vi "Wrap Data for UI Update.vi"(1 "References":T3, 2 "fpga inteface in":refnum<k20>, 3 "image metadata":T2={"serial channel"=0.0, "frame number"=0, "data type"=enum."Frame Start", "width"=0, "height"=0, "image bytes"=0, "total bytes"=0, "little endian"=FALSE, "Status"="Ready for Acquisition"}, 4 "Active Channel":string, 5 "error in":errorcluster) -> (7 "State message":string, 10 "Acqusition In Progress":bool, 11 "status":bool, 12 "Acquisition Duration":dbl, 14 "Image Data":string, 15 "Bytes Acquired":u64, 16 "PowerOverCoaxCurrent":dbl, 17 "PowerOverCoaxVoltage":dbl, 18 "width":u64, 19 "height":u64)   [LabVIEW 2025, in "Automotive Vision.lvclass"]
doc: "Wrap data for the measurement results cluster."
uses:
  Automotive Vision.lvclass
  Automotive Vision.lvclass/Automotive Vision.ctl
  <instrlib>/FlexRIO/CSI-2/v2/Common/Types/LLP Data Type.ctl
  <instrlib>/FlexRIO/CSI-2/v2/Common/NI CSI-2 API Common v2.lvlib
  <resource>/objmgr/niflexrioapiChannel.rc
  <instrlib>/FlexRIO/API/Host/v1/NI FlexRIO API v1.lvlib
  <instrlib>/FlexRIO/API/Host/v1/NI FlexRIO/API/Get Property Reference - Fpga Small.vi
panel:
  out "error out":errorcluster
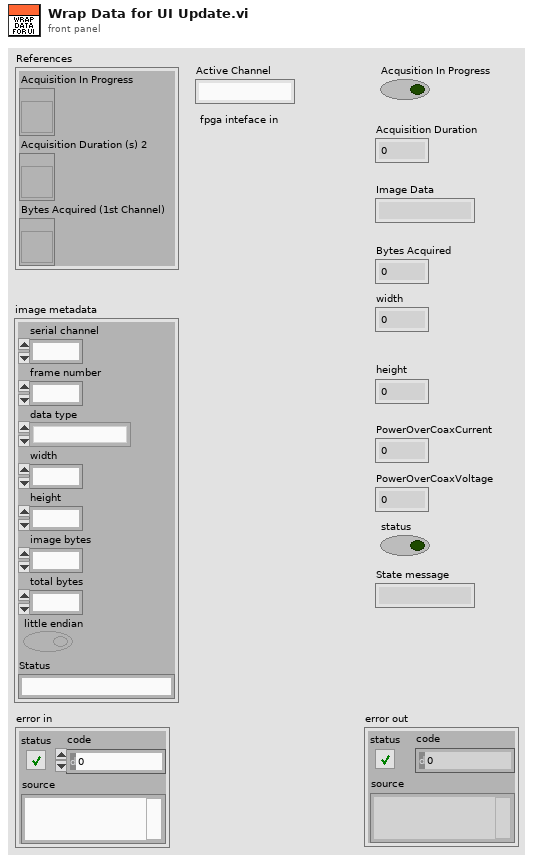
[diagram p1: front panel]
types:
  T1 = typedef "NI CSI-2 API Common v2.lvlib/LLP Data Type.ctl" = enum8{"Frame Start", "Frame End", "Line Start", "Line End", "End of Transmission", "Reserved 0", "Reserved 1", "Reserved 2", "Generic Short Packet 1", "Generic Short Packet 2", "Generic Short Packet 3", "Generic Short Packet 4", "Generic Short Packet 5", "Generic Short Packet 6", "Generic Short Packet 7", "Generic Short Packet 8", "Null", "Blanking Data", "Embedded 8-bit non Image Data", "Generic Long Packet 1", "Generic Long Packet 2", "Generic Long Packet 3", "Generic Long Packet 4", "Reserved 3", "YUV420 8-bit", "YUV420 10-bit", "Legacy YUV420 8-bit", "Reserved 4", "YUV420 8-bit Chroma Shifted", "YUV420 10-bit Chroma Shifted", "YUV422 8-bit", "YUV422 10-bit", "RGB444", "RGB555", "RGB565", "RGB666", "RGB888", "Reserved 5", "Reserved 6", "RAW 24", "RAW 6", "RAW 7", "RAW 8", "RAW 10", "RAW 12", "RAW 14", "RAW 16", "RAW 20", "User Defined 8-bit Data 1", "User Defined 8-bit Data 2", "User Defined 8-bit Data 3", "User Defined 8-bit Data 4", "User Defined 8-bit Data 5", "User Defined 8-bit Data 6", "User Defined 8-bit Data 7", "User Defined 8-bit Data 8", "USL Command", "Reserved 7", "Reserved 8", "Reserved 9", "Reserved 10", "Reserved 11", "Reserved 12", "LRTE EPD Spacer"}
  T2 = cluster{"serial channel":fxp<+,3,3>, "frame number":u16, "data type":T1, "width":u16, "height":u16, "image bytes":u32, "total bytes":u32, "little endian":bool, "Status":string}
  T3 = cluster{"Acquisition In Progress":refnum<vi>, "Acquisition Duration (s) 2":refnum<vi>, "Bytes Acquired (1st Channel)":refnum<vi>}
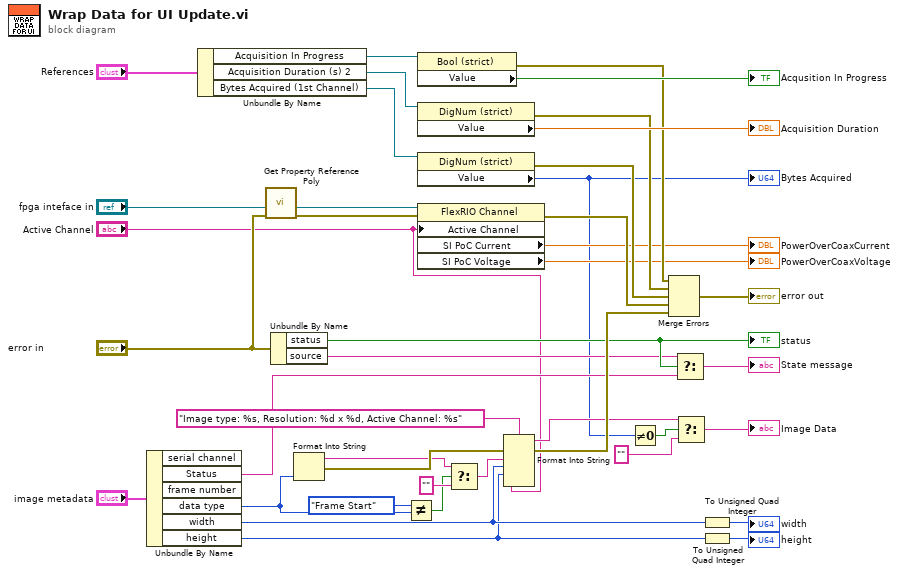
[diagram p0: block diagram]
diagram:
  n1 = Unbundle By Name("image metadata") -> ("Status"=w18:string, "data type"=w24:T1, "width"=w16:u16, "height"=w15:u16)  [unwired: 2 out]
  n2 = Unbundle By Name("References") -> ("Acquisition In Progress"=w34:refnum<vi>, "Acquisition Duration (s) 2"=w36:refnum<vi>, "Bytes Acquired (1st Channel)"=w38:refnum<vi>)
  n3 = call-poly <instrlib>:"Get Property Reference Poly.vi"("error in (no error)"="error in", "fpga interface in"="fpga inteface in") -> ("error out"=w7:errorcluster, "property reference"=w9:refnum<k20>)  [unwired: 4 in, 1 out]
  n4 = Unbundle By Name("error in") -> ("status"=w27:bool, "source"=w26:string)
  "status" <- w27
  n5 = Format Into String(w24) -> (resulting string=w22:string, error out=w30:errorcluster)  [unwired: 3 in]
  n6 = Not Equal?(x=LLP_Data_Type."Frame Start", y=w24) -> (x != y?=w19:bool)
  n7 = property on="Property Node" class="Bool (strict)"(reference=w34) -> (error out=w33:errorcluster, "Value"=→"Acqusition In Progress":bool)  [unwired: 1 in, 1 out]
  n8 = property on="Property Node" class="DigNum (strict)"(reference=w36) -> (error out=w32:errorcluster, "Value"=→"Acquisition Duration":dbl)  [unwired: 1 in, 1 out]
  n9 = property on="Property Node" class="DigNum (strict)"(reference=w38) -> (error out=w31:errorcluster, "Value"=w4:i64)  [unwired: 1 in, 1 out]
  "Bytes Acquired" <- w4
  n10 = property on="Property Node" class="FlexRIO Channel"(reference=w9, error in=w7, "Active Channel"="Active Channel") -> (error out=w13:errorcluster, "SI PoC Current"=→"PowerOverCoaxCurrent":dbl, "SI PoC Voltage"=→"PowerOverCoaxVoltage":dbl)  [unwired: 1 out]
  n11 = Select(t=w22, s=w19, f="") -> (s? t:f=w21:string)
  n12 = Format Into String(format string="Image type: %s, Resolution: %d x %d, Active Channel: %s", error in=w30, w21, w16, w15, "Active Channel") -> (resulting string=w6:string, error out=w29:errorcluster)  [unwired: 1 in]
  n13 = Not Equal To 0?(x=w4) -> (x != 0?=w5:bool)
  n14 = Merge Errors(w33, w32, w31, w13, w29) -> (→"error out":errorcluster)
  n15 = Select(t=w26, s=w27, f=w18) -> (s? t:f=→"State message":string)
  n16 = Select(t=w6, s=w5, f="") -> (s? t:f=→"Image Data":string)
  n17 = To Unsigned Quad Integer(1:w16) -> (0:→"width":u64)
  n18 = To Unsigned Quad Integer(1:w15) -> (0:→"height":u64)
